vi "UE9 Update DACs Example.vi"() -> ()   [LabVIEW 2021]
panel:
  in  "Binary":bool
  in  "DAC1":dbl format="%.4f"
  in  "DAC0":dbl format="%.4f"
  out "Error Message":string
  out "error out":errorcluster
  # "Updates both DACs over USB on the first found UE9."
  # "Volts, unless binary option is selected."
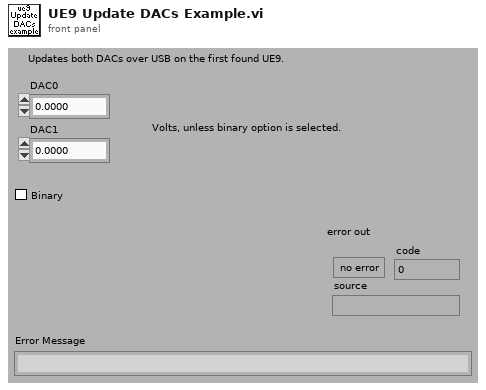
[diagram p1: front panel]
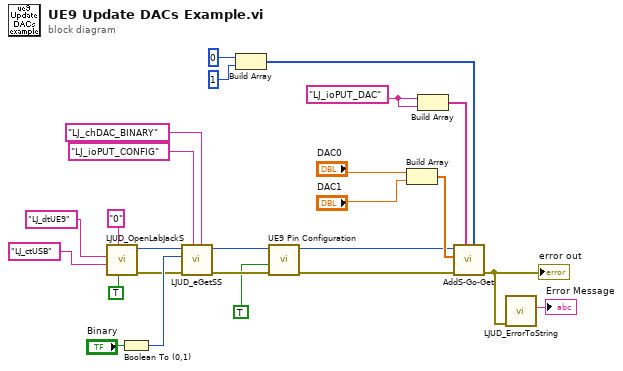
[diagram p0: block diagram]
diagram:
  w6 = "LJ_ioPUT_DAC" ("IOType")
  n1 = call "LJUD_OpenLabJackS.vi"("FirstFound"=TRUE, "Address"="0", "ConnectionType"="LJ_ctUSB", "DeviceType"="LJ_dtUE9") -> ("error out"=w11:errorcluster, "Handle"=w7:i32)  [unwired: 5 in, 1 out]
  n2 = Boolean To (0,1)(Boolean="Binary") -> (0, 1=w15:i16)
  n3 = call "LJUD_eGetSS.vi"("Channel"="LJ_chDAC_BINARY" ("IOType"), "IOType"="LJ_ioPUT_CONFIG", "error in"=w11, "Value Write"=w15, "Handle In"=w7) -> ("error out"=w4:errorcluster, "Handle Out"=w5:i32)  [unwired: 4 in, 1 out]
  n4 = Build Array(0 ("Input Element"), 1 ("Input Element")) -> (w18:i32[])
  n5 = call "UE9 Pin Configuration.vi"("error in"=w4, "Enable DACs"=TRUE, "Handle In"=w5) -> ("error out"=w2:errorcluster, "Handle Out"=w3:i32)  [unwired: 7 in]
  n6 = Build Array("DAC0", "DAC1") -> (w21:dbl[])
  n7 = Build Array(w6, w6) -> (w17:string[])
  n8 = call "AddS-Go-Get.vi"("Channels"=w18, "IOTypes"=w17, "error in"=w2, "Values Write"=w21, "Handle In"=w3) -> ("error out"=w24:errorcluster)  [unwired: 4 in, 2 out]
  "error out" <- w24
  n9 = call "LJUD_ErrorToString.vi"("error in"=w24) -> ("String"=→"Error Message":string)  [unwired: 10 in]
